vi "websocket control.vi"() -> ()   [LabVIEW 2014]
panel:
  in  "stop":bool
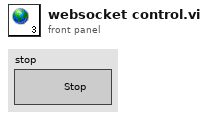
[diagram p1: front panel]
diagram:
